vi "GetCorruptedTics.vi"(11 "packet in":u8[](array[numeric])) -> (3 "corrupted ticks":u8)   [LabVIEW 2018]
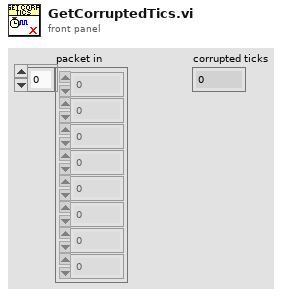
[diagram p1: front panel]
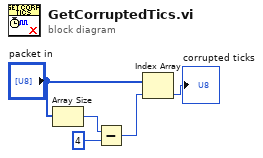
[diagram p0: block diagram]
diagram:
  n1 = Array Size(array="packet in") -> (size(s)=w1:i32)
  n2 = Subtract(x=w1, y=4) -> (x-y=w3:i32)
  n3 = Index Array(array="packet in", index=w3) -> (element=→"corrupted ticks":u8)
